vi "Decoder.vi"() -> ()   [LabVIEW 2016]
uses:
  <vilib>/rvi/Emulation/niFpgaGetClockAttributes.vi
  <vilib>/rvi/Emulation/niFpgaSctlEmulationGetInTimedLoop.vi
  <vilib>/rvi/Emulation/niFpgaEmulationReportErrorSimple.vi
  <vilib>/rvi/eio/common/nirviEmuTemplateMethod_errors.vi
  <vilib>/rvi/Emulation/niFpgaCriticalErrorInLSC.vi
  <vilib>/eio/EIONode/EIONode.xnode
  <vilib>/LabVIEW Targets/FPGA/RIO/nicrio_985x_controls.llb/CAN_IO_Frame Cluster.ctl
  <vilib>/LabVIEW Targets/FPGA/RIO/nicrio_985x_controls.llb/CAN_IO_Frame Type.ctl
panel:
  out "Motor power":u8
  out "Ready to drive":bool
  out "cooling liquid temperature":u8
  out "brake pedal position":u8
  out "accelerator position":u8
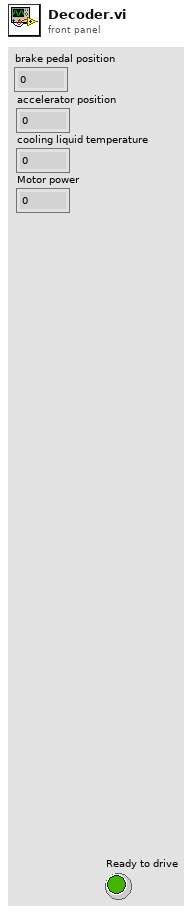
[diagram p1: front panel]
types:
  T1 = typedef "CAN_IO_Frame Cluster.ctl" = cluster{"timestamp high":u32, "timestamp low":u32, "identifier":u32, "type":T2, "info A":u8, "info B":u8, "data length":u8, "data":u8[]}
  T2 = typedef "CAN_IO_Frame Type.ctl" = enum8{"Data Frame", "Remote Frame", "(reserved)", "(reserved) ", "(reserved)  ", "(reserved)   ", "Bus Error", "Transceiver Fault"}
  T3 = cluster{"data[0]":u8, "data[1]":u8, "data[2]":u8, "data[3]":u8, "data[4]":u8, "data[5]":u8, "data[6]":u8, "data[7]":u8, "data[8]":u8}
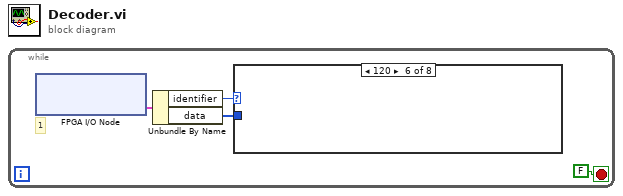
[diagram p0: block diagram]
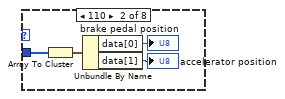
[diagram p3: hidden frame]
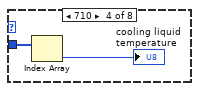
[diagram p5: hidden frame]
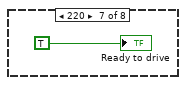
[diagram p7: hidden frame]
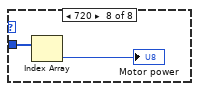
[diagram p8: hidden frame]
diagram:
  n1 = while {
    stop <- FALSE stop-if-true
    # "1"
    n2 = xnode "FPGA I/O Node"() -> ("Mod1/CAN1"=w3:T1)  [unwired: 2 in, 2 out]
    n3 = Unbundle By Name(w3) -> ("identifier"=w2:u32, "data"=w1:u8[])
    n4 = case shown="120" w2 {
      tunnel: w1 -> [_ w8 _ w10 _ _ _ w13]
      frame Default {
      }
      frame 110 {
        n5 = Array To Cluster(array=w8) -> (cluster=w7:T3)
        n6 = Unbundle By Name(w7) -> ("data[0]"=→"brake pedal position":u8, "data[1]"=→"accelerator position":u8)
      }
      frame 10 {
      }
      frame 710 {
        n7 = Index Array(array=w10) -> (element=→"cooling liquid temperature":u8)  [unwired: 1 in]
      }
      frame 90 {
      }
      frame 120 {
      }
      frame 220 {
        "Ready to drive" <- TRUE ("Ready to drive")
      }
      frame 720 {
        n8 = Index Array(array=w13) -> (element=→"Motor power":u8)  [unwired: 1 in]
      }
    }
  }
